vi "PRN Read_1.vi"(6 "Barcode Selection":u16(ring) items=["TSC -TA-345", "Zebra GC420t"], 9 "Model name":string, 10 "Serial no":string="zre") -> (0 "Pint Barcode":string, 2 "result string":string)   [LabVIEW 2015]
panel:
  out "result string 2":string
  out "offset past replacement":i32
  out "number of replacements":i32
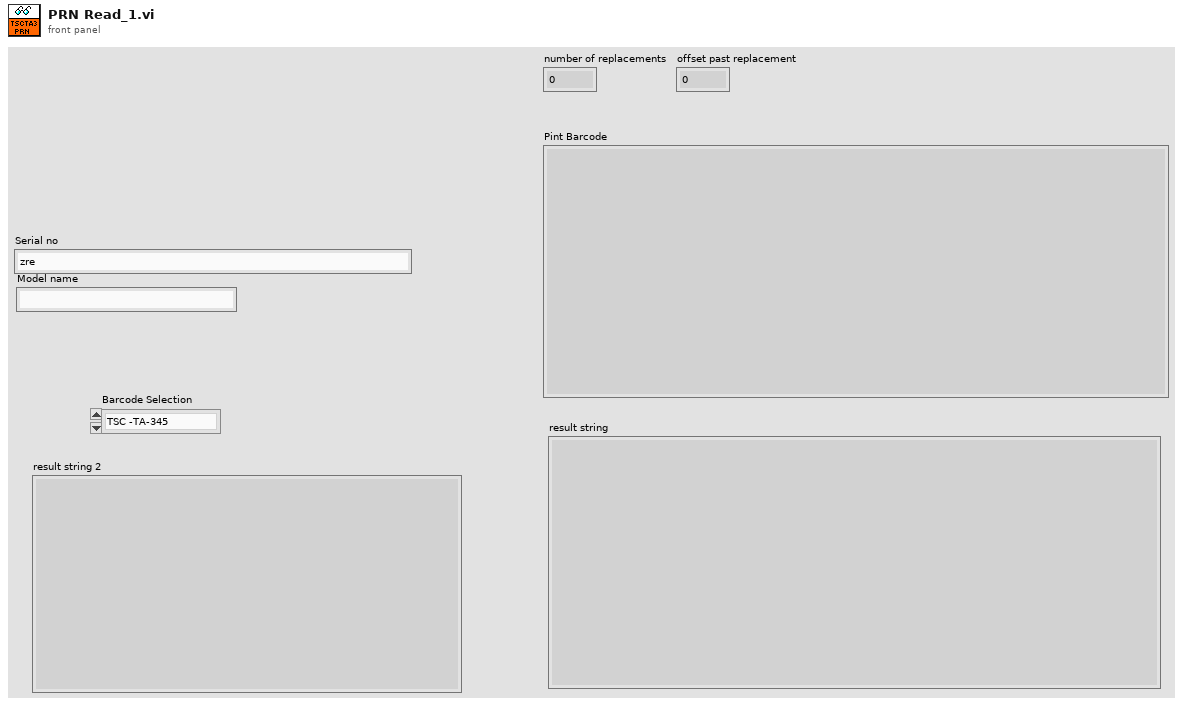
[diagram p1: front panel]
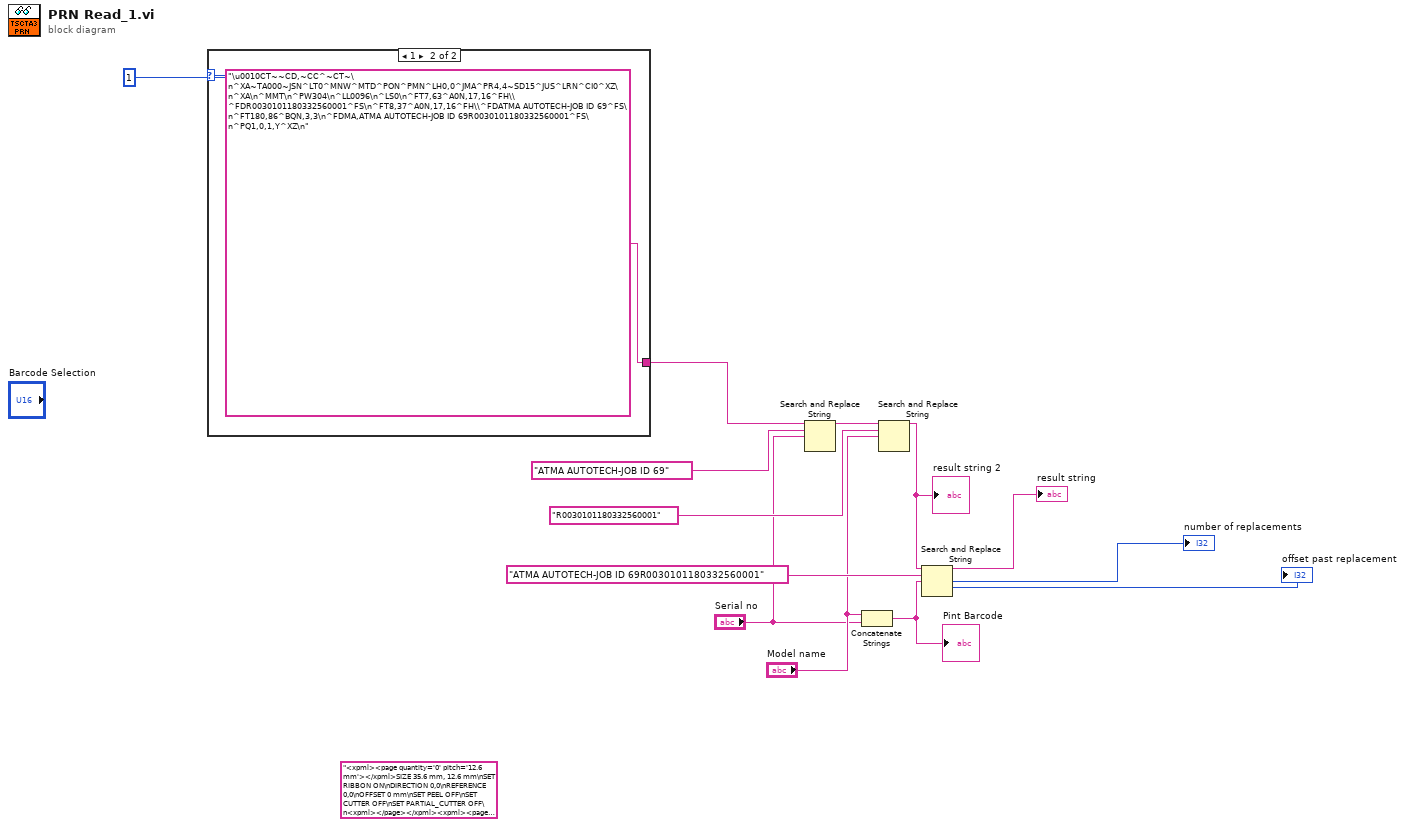
[diagram p0: block diagram]
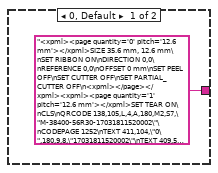
[diagram p2: hidden frame]
diagram:
  (unwired) "<xpml><page quantity='0' pitch='12.6 mm'></xpml>SIZE 35.6 mm, 12.6 mm\nSET RIBBON ON\nDIRECTION 0,0\nREFERENCE 0,0\nOFFSET 0 mm\nSET PEEL OFF\nSET CUTTER OFF\nSET PARTIAL_CUTTER OFF\n<xpml></page></xpml><xpml><page quantity='1' pitch='12.6 mm'></xpml>SET TEAR ON\nCLS\nQRCODE 89,91,L,4,A,180,M2,S7,\"M-38400-56R30-17031811520002\"\nCODEPAGE 1252\nTEXT 402,83,\"0\",180,8,8,\"17031811520002\"\nTEXT 402,42,\"0\",180,8,8,\"M-38400-56R30\"\nPRINT 1,1\n<xpml></page></xpml><xpml><end/></xpml>" ("write buffer")
  n1 = case shown="1" u16 1 {
    tunnel: ["<xpml><page quantity='0' pitch='12.6 mm'></xpml>SIZE 35.6 mm, 12.6 mm\nSET RIBBON ON\nDIRECTION 0,0\nREFERENCE 0,0\nOFFSET 0 mm\nSET PEEL OFF\nSET CUTTER OFF\nSET PARTIAL_CUTTER OFF\n<xpml></page></xpml><xpml><page quantity='1' pitch='12.6 mm'></xpml>SET TEAR ON\nCLS\nQRCODE 138,105,L,4,A,180,M2,S7,\"M-38400-56R30-17031811520002\"\nCODEPAGE 1252\nTEXT 411,104,\"0\",180,9,8,\"17031811520002\"\nTEXT 409,56,\"0\",180,9,8,\"M-38400-56R30\"\nPRINT 1,1\n<xpml></page></xpml><xpml><end/></xpml>" ("write buffer") "\u0010CT~~CD,~CC^~CT~\n^XA~TA000~JSN^LT0^MNW^MTD^PON^PMN^LH0,0^JMA^PR4,4~SD15^JUS^LRN^CI0^XZ\n^XA\n^MMT\n^PW304\n^LL0096\n^LS0\n^FT7,63^A0N,17,16^FH\\^FDR0030101180332560001^FS\n^FT8,37^A0N,17,16^FH\\^FDATMA AUTOTECH-JOB ID 69^FS\n^FT180,86^BQN,3,3\n^FDMA,ATMA AUTOTECH-JOB ID 69R0030101180332560001^FS\n^PQ1,0,1,Y^XZ\n"] -> w4
    frame 0, Default {
    }
    frame 1 {
    }
  }
  n2 = Search and Replace String(input string=w4, search string="ATMA AUTOTECH-JOB ID 69", replace string="Serial no") -> (result string=w6:string)  [unwired: 5 in, 3 out]
  n3 = Concatenate Strings("Model name", "Serial no") -> (w7:string)
  "Pint Barcode" <- w7
  n4 = Search and Replace String(input string=w6, search string="R0030101180332560001" ("replace string (\"\")"), replace string="Model name") -> (result string=w11:string)  [unwired: 5 in, 3 out]
  "result string 2" <- w11
  n5 = Search and Replace String(input string=w11, search string="ATMA AUTOTECH-JOB ID 69R0030101180332560001" ("replace string (\"\")"), replace string=w7) -> (result string=→"result string":string, number of replacements=→"number of replacements":i32, offset past replacement=→"offset past replacement":i32)  [unwired: 5 in, 1 out]
